vi "VIName.vi"(10 "error in (no error)":errorcluster, 11 "VI in":refnum<vi>) -> (0 "Name":string, 2 "error out":errorcluster, 3 "VI out":refnum<vi>)   [LabVIEW 2017, in "TagDB RefManager.lvlib"]
uses:
  TagDB RefManager.lvlib
  <userlib>/_NEVSTOP/TagDB/TagDB.lvlib
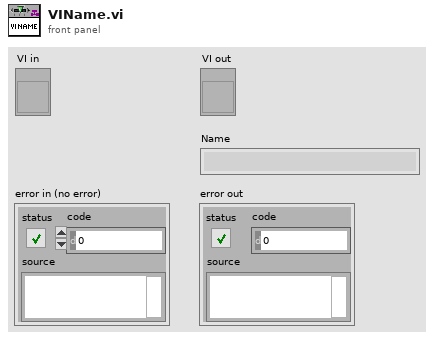
[diagram p1: front panel]
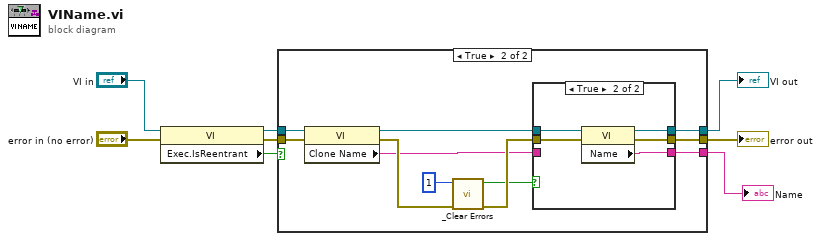
[diagram p0: block diagram]
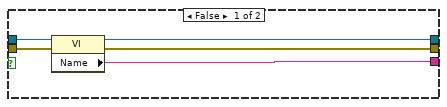
[diagram p2: hidden frame]
diagram:
  n1 = property on="Property Node" class="VI"(reference="VI in", error in="error in (no error)") -> (reference out=w5:refnum<vi>, error out=w6:errorcluster, "Exec.IsReentrant"=w8:bool)
  n2 = case shown="True" w8 {
    tunnel: [w11 w18] -> w1
    tunnel: [w10 w17] -> w2
    tunnel: [w9 w14] -> w3
    tunnel: w5 -> [w13 w23]
    tunnel: w6 -> [w12 w22]
    frame False {
      n3 = property class="VI"(reference=w13, error in=w12) -> (reference out=w11:refnum<vi>, error out=w10:errorcluster, "Name"=w9:string)
    }
    frame True {
      n4 = property class="VI"(reference=w23, error in=w22) -> (reference out=w20:refnum<vi>, error out=w24:errorcluster, "Clone Name"=w15:string)
      n5 = call <userlib>:"_Clear Errors.vi"("error in (no error)"=w24, "specific error code to clear (0: all)"=1) -> ("error out"=w19:errorcluster, "specific error cleared?"=w16:bool)  [unwired: 4 in]
      n6 = case shown="True" w16 {
        tunnel: w20 -> [w26 w32]
        tunnel: w19 -> [w25 w31]
        tunnel: [w26 w30] -> w18
        tunnel: [w25 w29] -> w17
        tunnel: w15 -> [w27 _]
        tunnel: [w27 w28] -> w14
        frame False {
        }
        frame True {
          n7 = property class="VI"(reference=w32, error in=w31) -> (reference out=w30:refnum<vi>, error out=w29:errorcluster, "Name"=w28:string)
        }
      }
    }
  }
  "Name" <- w3
  "error out" <- w2
  "VI out" <- w1
